vi "NaN_screening_big.vi"(11 "Input":T1 {"File Location" items=["Unknown"=-1, "Processing"=0, "Storage"=1]}) -> (3 "Output":T1 {"File Location" items=["Unknown"=-1, "Processing"=0, "Storage"=1]})   [LabVIEW 2013]
uses:
  User Interface/Controls/Post_Dust_Event.ctl
  User Interface/Controls/File_location.ctl
panel:
  # "Dust Event"
  # "Dust Event"
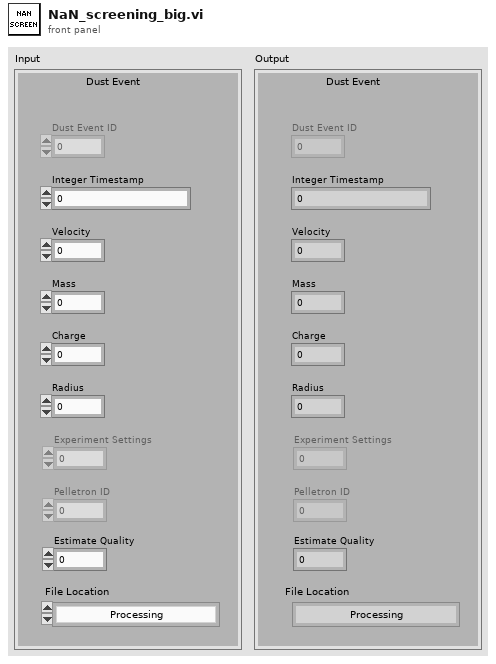
[diagram p1: front panel]
types:
  T1 = typedef "Post_Dust_Event.ctl" = cluster{"Dust Event ID":i64, "Integer Timestamp":i64, "Velocity":sgl, "Mass":sgl, "Charge":sgl, "Radius":sgl, "Experiment Settings":dbl, "Pelletron ID":i32, "Estimate Quality":sgl, "File Location":T2, "id_dust_info":dbl}
  T2 = typedef "File_location.ctl" = i8
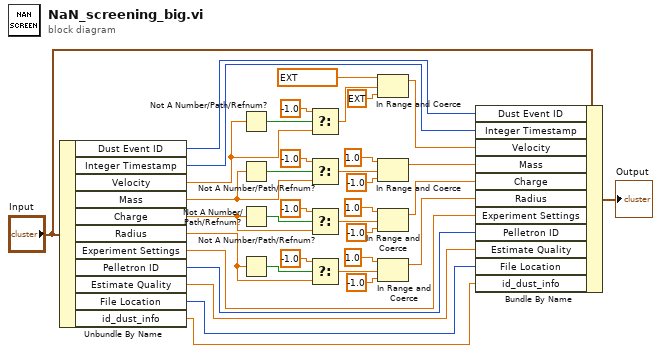
[diagram p0: block diagram]
diagram:
  n1 = Unbundle By Name("Input") -> ("Dust Event ID"=w35:i64, "Integer Timestamp"=w34:i64, "Velocity"=w22:sgl, "Mass"=w24:sgl, "Charge"=w26:sgl, "Radius"=w21:sgl, "Experiment Settings"=w33:dbl, "Pelletron ID"=w32:i32, "Estimate Quality"=w3:sgl, "File Location"=w2:T2, "id_dust_info"=w1:dbl)
  n2 = Not A Number/Path/Refnum?(number/path/refnum=w22) -> (NaN/Path/Refnum?=w23:bool)
  n3 = Not A Number/Path/Refnum?(number/path/refnum=w24) -> (NaN/Path/Refnum?=w25:bool)
  n4 = Not A Number/Path/Refnum?(number/path/refnum=w26) -> (NaN/Path/Refnum?=w28:bool)
  n5 = Not A Number/Path/Refnum?(number/path/refnum=w21) -> (NaN/Path/Refnum?=w20:bool)
  n6 = Select(t=-1.0 ("y"), s=w23, f=w22) -> (s? t:f=w17:dbl)
  n7 = Select(t=-1.0 ("y"), s=w25, f=w24) -> (s? t:f=w13:dbl)
  n8 = Select(t=-1.0 ("y"), s=w28, f=w26) -> (s? t:f=w7:dbl)
  n9 = Select(t=-1.0 ("y"), s=w20, f=w21) -> (s? t:f=w5:dbl)
  n10 = In Range and Coerce(upper limit=ext 299792458.0, x=w17, lower limit=ext -1.0) -> (coerced(x)=w16:ext)  [unwired: 1 out]
  n11 = In Range and Coerce(upper limit=1.0, x=w13, lower limit=-1.0) -> (coerced(x)=w12:dbl)  [unwired: 1 out]
  n12 = In Range and Coerce(upper limit=1.0, x=w7, lower limit=-1.0) -> (coerced(x)=w6:dbl)  [unwired: 1 out]
  n13 = In Range and Coerce(upper limit=1.0, x=w5, lower limit=-1.0) -> (coerced(x)=w4:dbl)  [unwired: 1 out]
  n14 = Bundle By Name(cluster="Input", "Dust Event ID"=w35, "Integer Timestamp"=w34, "Velocity"=w16, "Mass"=w12, "Charge"=w6, "Radius"=w4, "Experiment Settings"=w33, "Pelletron ID"=w32, "Estimate Quality"=w3, "File Location"=w2, "id_dust_info"=w1) -> (→"Output":T1)
